vi "Configure FFT Phase Reference.vi"(8 "error in (no error)":errorcluster, 9 "Math Function Index (1: Math Function 1)":i32(ring)=1 items=["Math Function 1"=1, "Math Function 2"=2, "Math Function 3"=3, "Math Function 4"=4], 10 "Reference Point (0: Trigger)":i32(ring) items=["Trigger", "Display"], 11 "VISA resource name":refnum<visa-resource-name>) -> (0 "error out":errorcluster, 3 "VISA resource name out":refnum<visa-resource-name>)   [LabVIEW 2017, in "Agilent 2000 3000 X-Series.lvlib"]
doc: "Specifies the reference point for calculating the FFT phase function.\n\nNote:\nThis VI is only applicable for 3000T, 3000G, 4000, 6000, 1000 Series"
uses:
  Agilent 2000 3000 X-Series.lvlib
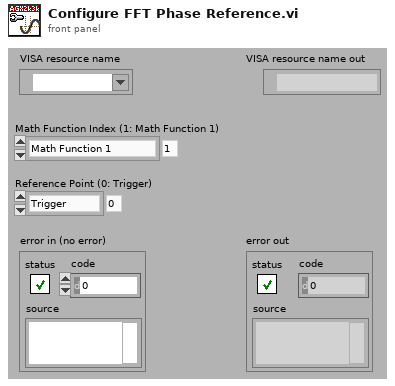
[diagram p1: front panel]
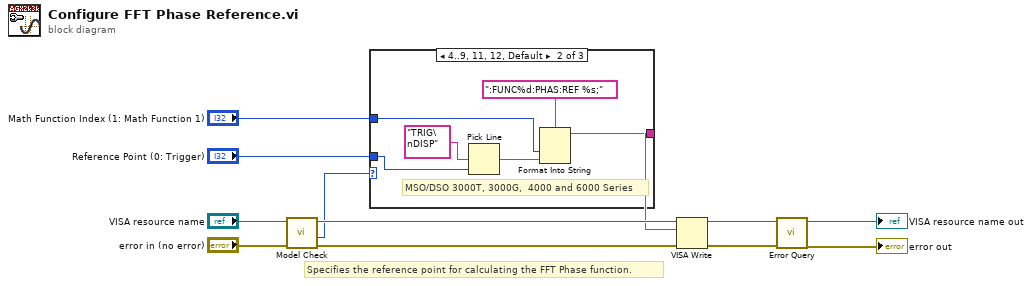
[diagram p0: block diagram]
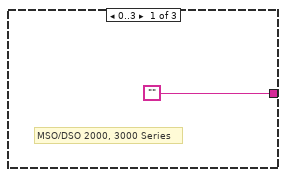
[diagram p2: hidden frame]
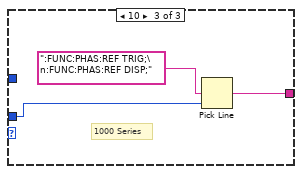
[diagram p3: hidden frame]
diagram:
  # "Specifies the reference point for calculating the FFT Phase function."
  n1 = call "Model Check.vi"("error in (no error)"="error in (no error)", "VISA resource name"="VISA resource name") -> ("error out"=w5:errorcluster, "Model"=w3:i32, "VISA resource name out"=w4:refnum<visa-resource-name>)  [unwired: 7 out]
  n2 = case shown="4..9, 11, 12, Default" w3 {
    tunnel: "Reference Point (0: Trigger)" -> [_ w15 w20]
    tunnel: ["" w14 w21] -> w2
    tunnel: "Math Function Index (1: Math Function 1)" -> [_ w17 _]
    frame 0..3 {
      # "MSO/DSO 2000, 3000 Series"
    }
    frame 4..9, 11, 12, Default {
      # "MSO/DSO 3000T, 3000G,  4000 and 6000 Series"
      n3 = Pick Line(multi-line string="TRIG\nDISP", line index=w15) -> (output string=w19:string)  [unwired: 1 in]
      n4 = Format Into String(format string=":FUNC%d:PHAS:REF %s;", w17, w19) -> (resulting string=w14:string)  [unwired: 2 in, 1 out]
    }
    frame 10 {
      # "1000 Series"
      n5 = Pick Line(multi-line string=":FUNC:PHAS:REF TRIG;\n:FUNC:PHAS:REF DISP;", line index=w20) -> (output string=w21:string)  [unwired: 1 in]
    }
  }
  n6 = VISA Write(VISA resource name=w4, write buffer=w2, error in (no error)=w5) -> (VISA resource name out=w11:refnum<visa-resource-name>, error out=w10:errorcluster)  [unwired: 1 out]
  n7 = call "Error Query.vi"("error in (no error)"=w10, "VISA resource name"=w11) -> ("error out"=→"error out":errorcluster, "VISA resource name out"=→"VISA resource name out":refnum<visa-resource-name>)  [unwired: 6 in, 2 out]
